vi "FG Vehicle ID.vi"(1 "FG Action (Read)":T1, 2 "Vehicle ID in":T2={"Subsystem Id"=90, "Node Id"=1, "Component Id"=1}) -> (0 "Vehicle ID out":T2={"Subsystem Id"=90, "Node Id"=1, "Component Id"=1})   [LabVIEW 2009]
uses:
  Address.ctl
  cRIO/Functional Global Variables/Actions for FG's.ctl
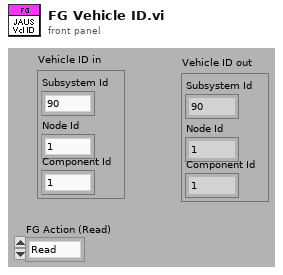
[diagram p1: front panel]
types:
  T1 = typedef "Actions for FG's.ctl" = enum16{"Read", "Write"}
  T2 = typedef "Address.ctl" = cluster{"Subsystem Id":u16, "Node Id":u8, "Component Id":u8}
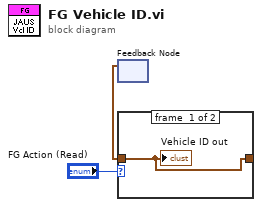
[diagram p0: block diagram]
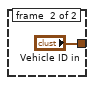
[diagram p2: hidden frame]
diagram:
  n1 = feedback #1() -> (w2:T2)  [unwired: 1 in]
  n2 = case shown="\"Write\"" "FG Action (Read)" {
    tunnel: w2 -> [w4 _]
    tunnel: [w4 "Vehicle ID in"] -> w3
    frame #0 {
      "Vehicle ID out" <- w4
    }
    frame #1 {
    }
  }
